vi "Initialize Transfer Groups.vi"(8 "error in (no error)":errorcluster, 9 "total # of Transfer Groups":i32, 10 "Transfer Groups":refnum<class "Transfer Group.lvclass">[](array[class]), 11 "Plugin Thread in":refnum<class "Plugin Thread.lvclass">) -> (0 "error out":errorcluster, 3 "Plugin Thread out":refnum<class "Plugin Thread.lvclass">)   [LabVIEW 2020, in "DSF Core.lvlib" / "Plugin Thread.lvclass"]
uses:
  Plugin Thread.lvclass
  Transfer Group/Transfer Group.lvclass
  Transfer Group/Transfer Group.lvclass/Transfer Group.ctl
  Plugin Thread.lvclass/Plugin Thread.ctl
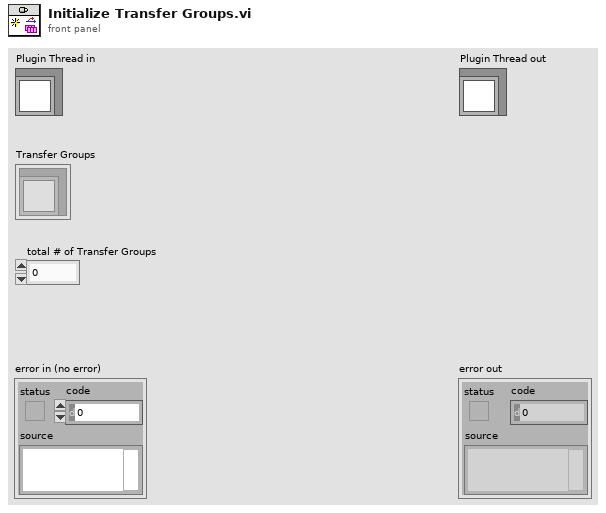
[diagram p1: front panel]
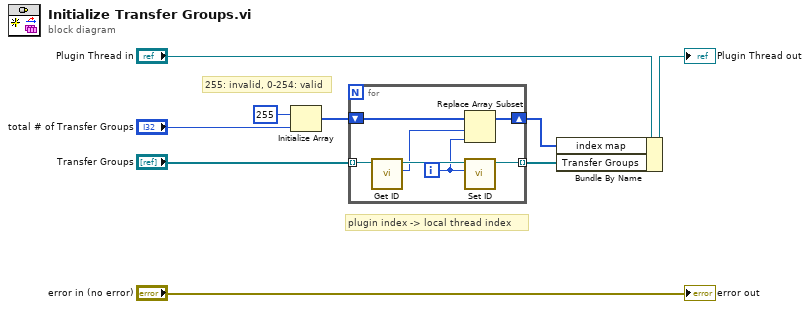
[diagram p0: block diagram]
diagram:
  # "255: invalid, 0-254: valid"
  # "plugin index -> local thread index"
  n1 = Initialize Array(u8 255 ("id"), "total # of Transfer Groups") -> (w3:u8[])
  n2 = for {
    tunnel: "Transfer Groups" -> [w16] mode=indexing
    tunnel: [w14] -> w6 mode=indexing
    shift-right: [w12] -> w2
    shift-left: w3 -> [w13]
    i -> [w10]
    n3 = call "Get ID.vi"("Transfer Group in"=w16) -> ("id"=w11:i32, "Transfer Group out"=w15:refnum<class "Transfer Group.lvclass">)  [unwired: 9 in]
    n4 = Replace Array Subset(array=w13, new element=w10, index=w11) -> (w12:u8[])
    n5 = call "Set ID.vi"("id"=w10, "Transfer Group in"=w15) -> ("Transfer Group out"=w14:refnum<class "Transfer Group.lvclass">)  [unwired: 9 in]
  }
  n6 = Bundle By Name(cluster="Plugin Thread in", "index map"=w2, "Transfer Groups"=w6) -> (→"Plugin Thread out":refnum<class "Plugin Thread.lvclass">)
  "error out" <- "error in (no error)"
